vi "Calibrate Moisture SLB.vi"(7 "GEA Inputs":T2={"Source"=228, "Destination"=36} {"Destination" format="%.0x"; "Source" format="%.0x"}, 8 "error in (no error)":errorcluster, 9 "Config File Path":path=path "C:/Automation/Configurations/JusticeLeague.ini", 10 "Desired Value Out":dbl=2400.0, 11 "Auto Cal State":T1) -> (0 "error out":errorcluster, 1 "GEA2 Reference Out":refnum<k24>, 2 "Report Text":string, 3 "Pass/Fail?":bool)   [LabVIEW 2016]
uses:
  Common/LabVIEW GEA2 Toolkit/LabVIEW_GEA2_Toolkit.lvlibp/type defs/Source_Destination.ctl
  Type Defs/JL_FMV Cal Action.ctl
  Q:/Common/DLLs/GEA3/GeaCommunication.dll
  Common/DLLs/GEA3/GeaCommunication.dll
  Common/LabVIEW GEA2 Toolkit/LabVIEW_GEA2_Toolkit.lvlibp/type defs/ERD Read Data In.ctl
  Common/LabVIEW GEA2 Toolkit/LabVIEW_GEA2_Toolkit.lvlibp/type defs/Data Type.ctl
  DAQ/Controls/Moisture Data.ctl
  Tools/Laundry/JL Dryer Tool/JL Dryer Tool Support/UTL_JL Scaling Factor Folder/Controls/ENUM_JL Scaling Factor_.ctl
  Common/LabVIEW GEA2 Toolkit/LabVIEW_GEA2_Toolkit.lvlibp
panel:
  out "Elapsed Time (s)":dbl
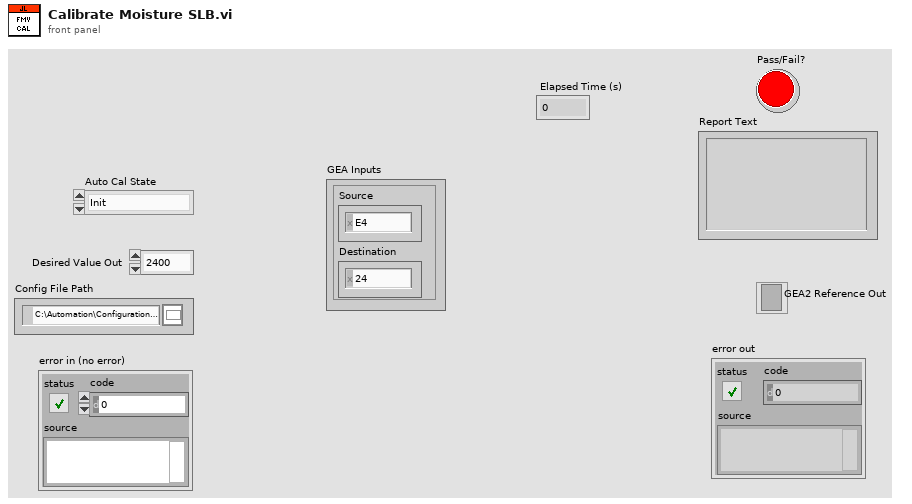
[diagram p1: front panel]
types:
  T1 = typedef "JL_FMV Cal Action.ctl" = enum16{"Init", "Reset Moisture", "Set Voltage Dither", "Wait", "Read GEA2", "Cal Low ", "Cal High", "Set Desired Moisture", "Flush Slope", "Save Cal ", "Exit"}
  T2 = typedef "LabVIEW_GEA2_Toolkit.lvlibp/Source_Destination.ctl" = cluster{"Source":u8, "Destination":u8}
  T3 = typedef "LabVIEW_GEA2_Toolkit.lvlibp/ERD Read Data In.ctl" = cluster{"ERD Number":u16, "Data Type":T4}
  T4 = typedef "LabVIEW_GEA2_Toolkit.lvlibp/Data Type.ctl" = enum16{"string", "boolean", "uint8_t", "uint16_t", "uint32_t", "uint64_t", "int8_t", "int16_t", "int32_t", "int64_t"}
  T5 = typedef "Moisture Data.ctl" = cluster{"Moisture (V)":dbl, "Dither":dbl, "Stop":bool}
  T6 = typedef "ENUM_JL Scaling Factor_.ctl" = enum16{"Init", "Scale Voltage", "Flush Slope"}
  T7 = cluster{"Raw Low ":dbl, "Raw High":dbl, "Actual Low":dbl, "Actual High":dbl}
  T8 = cluster{"Calibrate?":bool, "Scalling In ":cluster{"Raw Low ":dbl, "Raw High":dbl, "Actual Low":dbl, "Actual High":dbl}}
  T9 = typedef "LabVIEW_GEA2_Toolkit.lvlibp/ERD Read Data Out.ctl" = cluster{"ERD Number":u16, "Data":string}
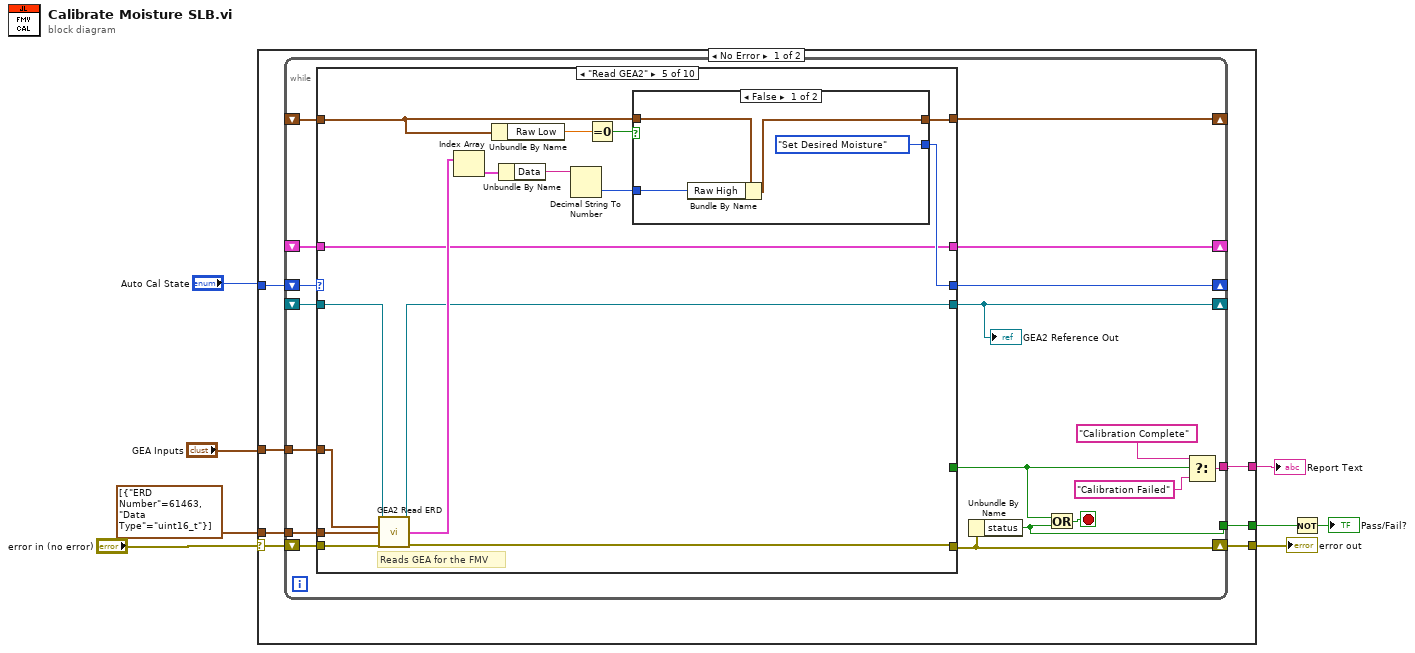
[diagram p0: block diagram]
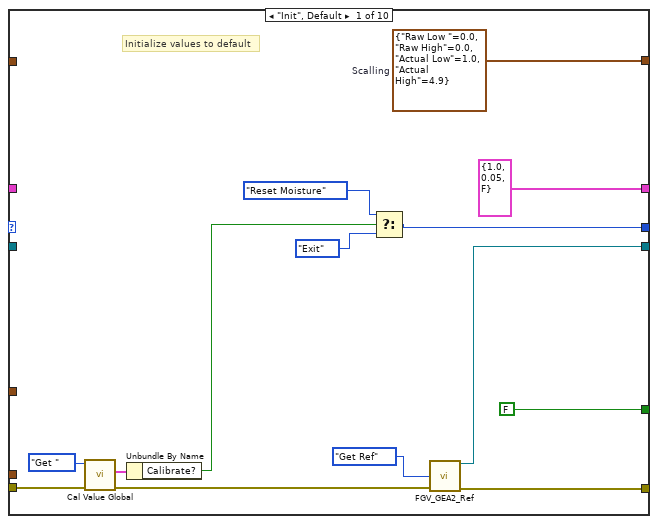
[diagram p2: hidden frame]
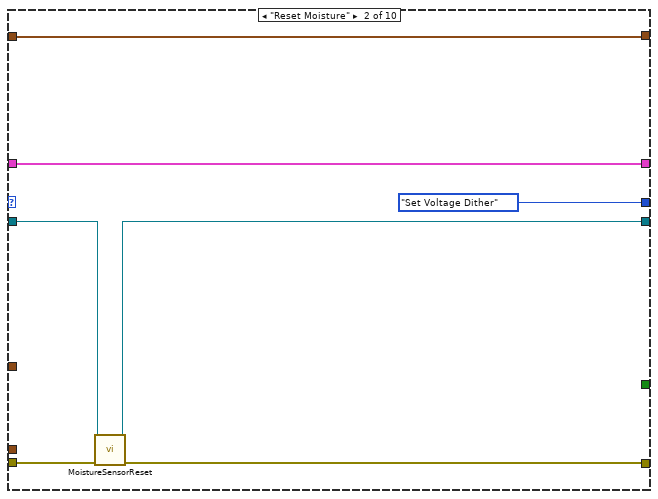
[diagram p3: hidden frame]
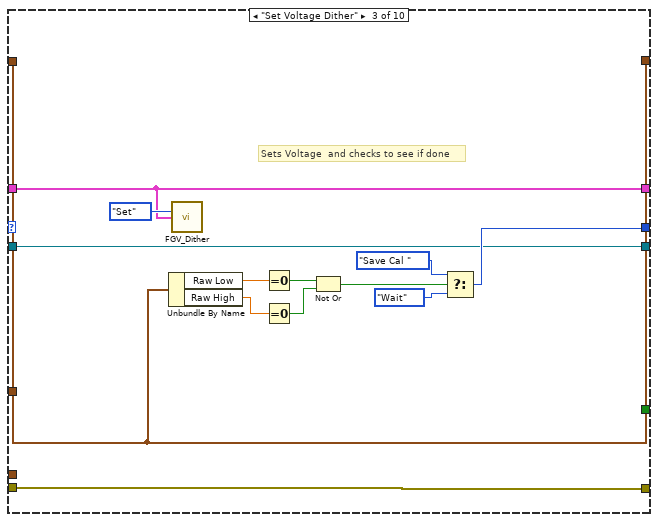
[diagram p4: hidden frame]
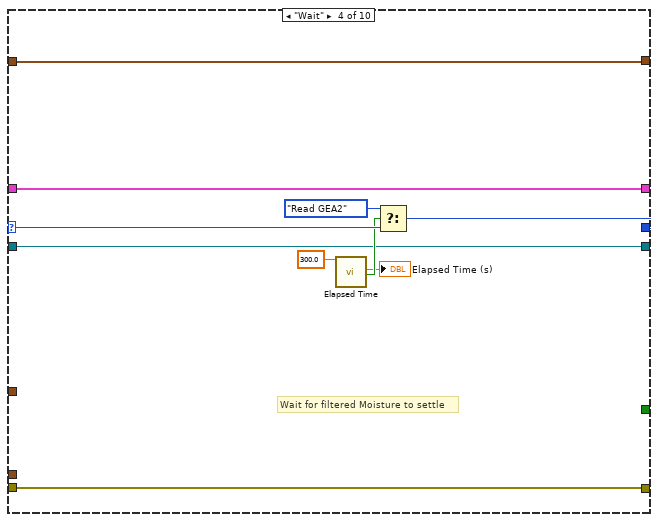
[diagram p5: hidden frame]
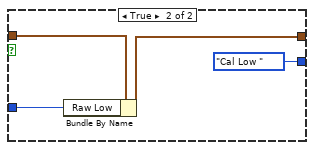
[diagram p6: hidden frame]
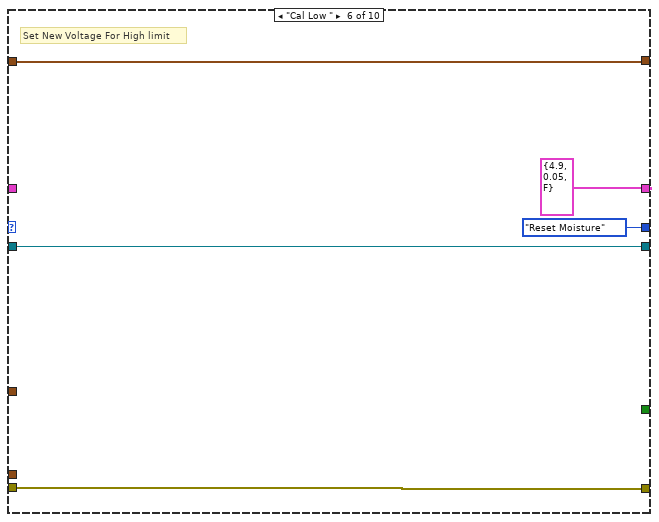
[diagram p7: hidden frame]
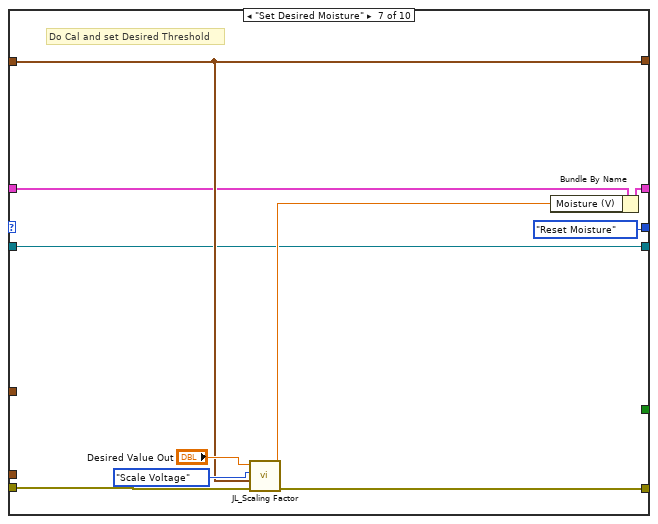
[diagram p8: hidden frame]
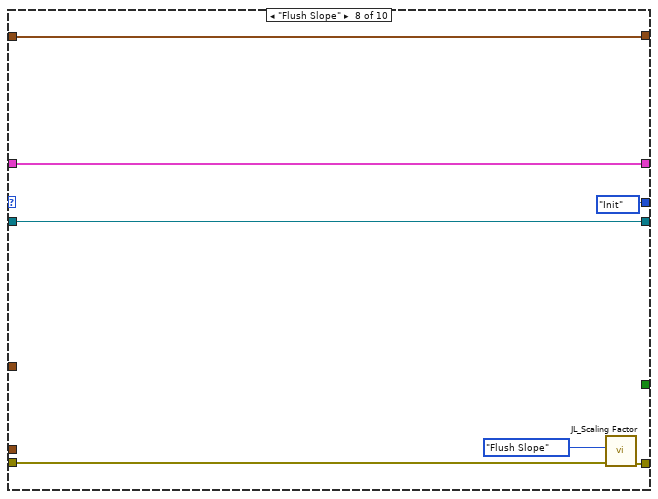
[diagram p9: hidden frame]
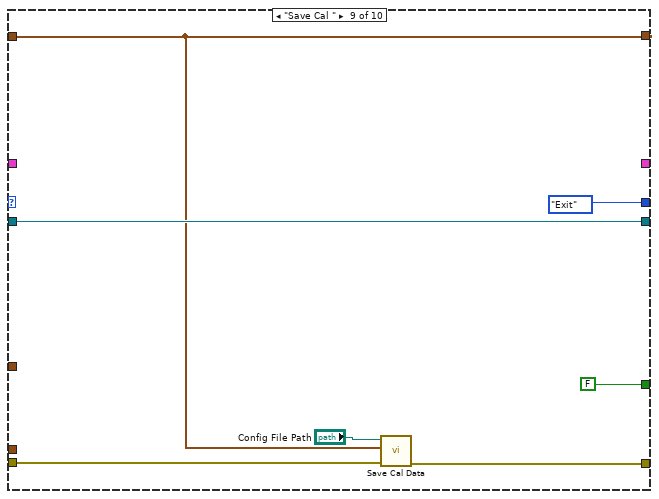
[diagram p10: hidden frame]
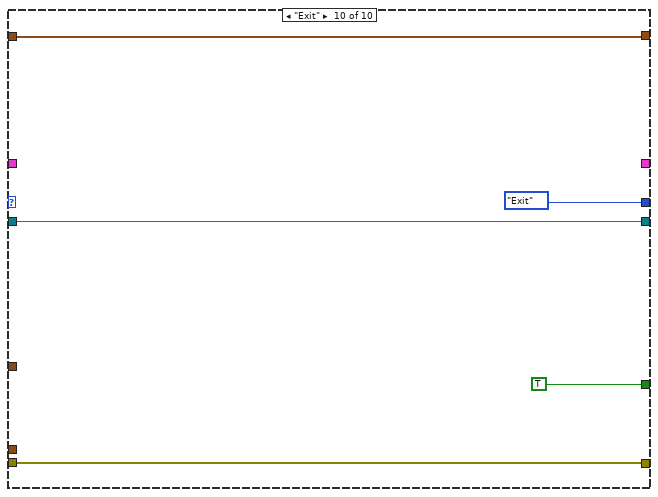
[diagram p11: hidden frame]
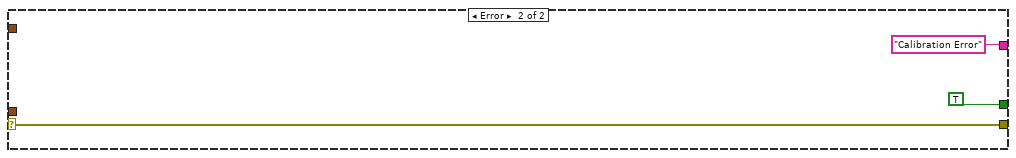
[diagram p12: hidden frame]
diagram:
  n1 = case shown="No Error" "error in (no error)" {
    selector: "error in (no error)" -> [w15 w138]
    tunnel: [w14 w138] -> w8
    tunnel: [w13 "Calibration Error" ("f")] -> w7
    tunnel: [w12 TRUE ("status")] -> w5
    tunnel: "Auto Cal State" -> [w11 _]
    tunnel: T3[] [{"ERD Number"=61463, "Data Type"=enum."uint16_t"}] ("Read ERD List") -> [w10 _]
    tunnel: "GEA Inputs" -> [w9 _]
    frame No Error {
      n2 = while {
        shift-right: [w33] -> _
        shift-left: _ -> [w28]
        shift-right: [w32] -> _
        shift-left: w11 -> [w31]
        shift-right: [w30] -> _
        shift-left: _ -> [w29]
        tunnel: w9 -> [w27]
        tunnel: w10 -> [w26]
        shift-right: [w16] -> _
        shift-left: _ -> [w24]
        shift-right: [w23] -> w14
        shift-left: w15 -> [w25]
        tunnel: [w20] -> w13
        tunnel: [w18] -> w12
        stop <- w22 stop-if-true
        n3 = case shown="\"Read GEA2\"" w31 {
          selector: w31 -> [_ _ _ w76 _ _ _ _ _ _]
          tunnel: [w47 w53 w64 w71 w83 w104 w113 w123 w124 w133] -> w33
          tunnel: w24 -> [_ w54 w55 w68 w87 w102 w107 w117 w129 w132]
          tunnel: [w37 JL_FMV_Cal_Action."Set Voltage Dither" ("Auto Cal State") w59 w74 w84 JL_FMV_Cal_Action."Reset Moisture" ("Auto Cal State") JL_FMV_Cal_Action."Reset Moisture" ("Auto Cal State") JL_FMV_Cal_Action."Init" ("Auto Cal State") JL_FMV_Cal_Action."Exit" ("Auto Cal State") JL_FMV_Cal_Action."Exit" ("Auto Cal State")] -> w32
          tunnel: [T5 {"Moisture (V)"=1.0, "Dither"=0.05, "Stop"=FALSE} ("Moisture Data In") w51 w66 w73 w81 T5 {"Moisture (V)"=4.9, "Dither"=0.05, "Stop"=FALSE} ("Moisture Data In") w110 w122 _ _] -> w30
          tunnel: w29 -> [_ w51 w66 w73 w81 _ w111 w122 _ _]
          tunnel: w28 -> [_ w53 w64 w71 w82 w104 w113 w123 w124 w133]
          tunnel: [FALSE _ _ _ _ _ _ _ FALSE TRUE] -> w17
          tunnel: w27 -> [_ _ _ _ w90 _ _ _ _ _]
          tunnel: w26 -> [_ _ _ _ w88 _ _ _ _ _]
          tunnel: w25 -> [w35 w50 w56 w69 w80 w103 w109 w120 w127 w131]
          tunnel: [w42 w49 w56 w69 w79 w103 w108 w119 w126 w131] -> w23
          tunnel: [w43 w48 w55 w68 w78 w102 w107 w117 w129 w132] -> w16
          frame "Init", Default {
            w47 = T7 {"Raw Low "=0.0, "Raw High"=0.0, "Actual Low"=1.0, "Actual High"=4.9}  # Scalling
            # "Initialize values to default"
            n4 = call "Cal Value Global.vi"("error in (no error)"=w35, "Action"=enum16{"Set", "Get "}."Get ") -> ("error out"=w34:errorcluster, "Cal  Out"=w40:T8)  [unwired: 8 in]
            n5 = Unbundle By Name(w40) -> ("Calibrate?"=w36:bool)
            n6 = Select(t=JL_FMV_Cal_Action."Reset Moisture" ("Auto Cal State"), s=w36, f=JL_FMV_Cal_Action."Exit") -> (s? t:f=w37:T1)
            n7 = call "FGV_GEA2_Ref.vi"("Action"=enum16{"Set Ref", "Get Ref"}."Get Ref", "Error In"=w34) -> ("GEA2 Reference Out"=w43:refnum<k24>, "Error Out"=w42:errorcluster)  [unwired: 12 in]
          }
          frame "Reset Moisture" {
            n8 = call "MoistureSensorReset.vi"("GEA2 Reference In"=w54, "Error In"=w50) -> ("GEA2 Reference Out"=w48:refnum<k24>, "Error Out"=w49:errorcluster)  [unwired: 10 in, 2 out]
          }
          frame "Set Voltage Dither" {
            # "Sets Voltage  and checks to see if done"
            n9 = Unbundle By Name(w64) -> ("Raw Low"=w65:dbl, "Raw High"=w63:dbl)
            n10 = call "FGV_Dither.vi"("Action"=enum16{"Set", "Get "}."Set", "Moisture Data In"=w66) -> ()  [unwired: 12 in, 2 out]
            n11 = Equal To 0?(x=w65) -> (x = 0?=w62:bool)
            n12 = Equal To 0?(x=w63) -> (x = 0?=w61:bool)
            n13 = Not Or(1:w61, 2:w62) -> (0:w60:bool)
            n14 = Select(t=JL_FMV_Cal_Action."Save Cal " ("Auto Cal State"), s=w60, f=JL_FMV_Cal_Action."Wait" ("Auto Cal State")) -> (s? t:f=w59:T1)
          }
          frame "Wait" {
            # "Wait for filtered Moisture to settle"
            n15 = call "Elapsed Time"("Time Target (s)"=300.0) -> ("Elapsed Time (s)"=→"Elapsed Time (s)":dbl, "Time has Elapsed"=w75:bool)  [unwired: 11 in, 6 out]
            n16 = Select(t=JL_FMV_Cal_Action."Read GEA2" ("Auto Cal State"), s=w75, f=w76) -> (s? t:f=w74:T1)
          }
          frame "Read GEA2" {
            # "Reads GEA for the FMV"
            n17 = call "GEA2 Read ERD.vi"("GEA2 Reference In"=w87, "GEA Inputs"=w90, "Read ERD List"=w88, "Error In"=w80) -> ("GEA2 Reference Out"=w78:refnum<k24>, "ERD Data Out"=w89:T9[], "Error Out"=w79:errorcluster)  [unwired: 8 in, 1 out]
            n18 = Index Array(array=w89) -> (element=w92:T9)  [unwired: 1 in]
            n19 = Unbundle By Name(w82) -> ("Raw Low"=w93:dbl)
            n20 = Unbundle By Name(w92) -> ("Data"=w91:string)
            n21 = Decimal String To Number(string=w91) -> (number=w85:i32)  [unwired: 2 in, 1 out]
            n22 = Equal To 0?(x=w93) -> (x = 0?=w86:bool)
            n23 = case shown="False" w86 {
              tunnel: [w94 w98] -> w83
              tunnel: w85 -> [w96 w101]
              tunnel: [JL_FMV_Cal_Action."Set Desired Moisture" ("Auto Cal State") JL_FMV_Cal_Action."Cal Low " ("Auto Cal State")] -> w84
              tunnel: w82 -> [w95 w99]
              frame False {
                n24 = Bundle By Name(cluster=w95, "Raw High"=w96) -> (w94:T7)
              }
              frame True {
                n25 = Bundle By Name(cluster=w99, "Raw Low"=w101) -> (w98:T7)
              }
            }
          }
          frame "Cal Low " {
            # "Set New Voltage For High limit"
          }
          frame "Set Desired Moisture" {
            # "Do Cal and set Desired Threshold"
            n26 = call "JL_Scaling Factor.vi"("Error"=w109, "Scalling"=w113, "Scaling Type"=ENUM_JL_Scaling_Factor_."Scale Voltage", "Desired Value Out"="Desired Value Out") -> ("Error Out"=w108:errorcluster, "Analog Value Out"=w112:dbl)  [unwired: 5 in, 1 out]
            n27 = Bundle By Name(cluster=w111, "Moisture (V)"=w112) -> (w110:T5)
          }
          frame "Flush Slope" {
            n28 = call "JL_Scaling Factor.vi"("Error"=w120, "Scaling Type"=ENUM_JL_Scaling_Factor_."Flush Slope") -> ("Error Out"=w119:errorcluster)  [unwired: 7 in, 2 out]
          }
          frame "Save Cal " {
            n29 = call "Save Cal Data.vi"("Error In"=w127, "Scalling"=w124, "Config File Path"="Config File Path") -> ("error out"=w126:errorcluster)  [unwired: 8 in]
          }
          frame "Exit" {
          }
        }
        "GEA2 Reference Out" <- w16
        n30 = Unbundle By Name(w23) -> ("status"=w18:bool)
        n31 = Or(x=w17, y=w18) -> (x .or. y?=w22:bool)
        n32 = Select(t="Calibration Complete" ("Report Text"), s=w17, f="Calibration Failed") -> (s? t:f=w20:string)
      }
    }
    frame Error {
    }
  }
  "error out" <- w8
  "Report Text" <- w7
  n33 = Not(x=w5) -> (.not. x?=→"Pass/Fail?":bool)
